vi "GetRealExposureTime.vi"(8 "error in (no error)":errorcluster) -> (0 "error out":errorcluster, 3 "Actual Exposure Time (ms)":dbl)   [LabVIEW 2015]
uses:
  LiveImage_Global.vi
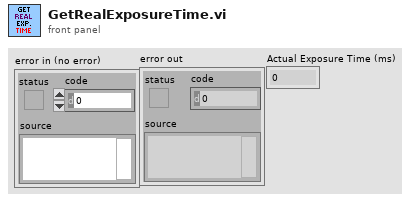
[diagram p1: front panel]
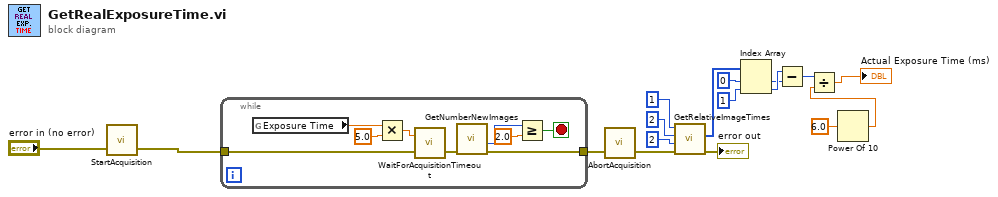
[diagram p0: block diagram]
diagram:
  n1 = call <userlib>:"StartAcquisition.vi"("error in (no error)"="error in (no error)") -> ("error out"=w16:errorcluster)  [unwired: 1 in, 1 out]
  n2 = while {
    tunnel: w16 -> [w26]
    tunnel: [w18] -> w13
    stop <- w19 stop-if-true
    n3 = global read "LiveImage_Global.vi" "Exposure Time"() -> (w25:dbl)
    n4 = Multiply(x=w25, y=5.0) -> (x*y=w23:dbl)
    n5 = call <userlib>:"WaitForAcquisitionTimeout.vi"("error in (no error)"=w26, "iTimeOutMs"=w23) -> ("error out"=w22:errorcluster)  [unwired: 1 out]
    n6 = call <userlib>:"GetNumberNewImages.vi"("error in (no error)"=w22) -> ("error out"=w18:errorcluster, "last"=w20:i32)  [unwired: 3 in, 2 out]
    n7 = Greater Or Equal?(x=w20, y=2.0) -> (x >= y?=w19:bool)
  }
  n8 = call <userlib>:"AbortAcquisition.vi"("error in (no error)"=w13) -> ("error out"=w12:errorcluster)  [unwired: 1 in, 1 out]
  n9 = call <userlib>:"GetRelativeImageTimes.vi"("error in (no error)"=w12, "size"=u32 2, "last"=u32 2, "first"=u32 1) -> ("error out"=→"error out":errorcluster, "arr"=w8:u64[])  [unwired: 5 in, 1 out]
  n10 = Index Array(array=w8, index #1=0 ("index"), index #2=1 ("index")) -> (element #1=w6:u64, element #2=w7:u64)
  n11 = Subtract(x=w7, y=w6) -> (x-y=w4:u64)
  n12 = Power Of 10(x=6.0) -> (10^x=w1:dbl)
  n13 = Divide(x=w4, y=w1) -> (x/y=→"Actual Exposure Time (ms)":dbl)
